vi "Fpga-Test-Harness.vi"() -> ()   [LabVIEW 2016]
uses:
  <vilib>/Platform/TimedLoop/XDataNode/timing_clust.ctl
  <vilib>/Platform/TimedLoop/XDataNode/nitl_modes.ctl
  <vilib>/Platform/TimedLoop/XDataNode/wakeup.ctl
  <vilib>/rvi/Emulation/niFpgaSctlEmulationGetInTimedLoop.vi
  <vilib>/rvi/Emulation/niFpgaEmulationReportErrorSimple.vi
  <vilib>/rvi/Emulation/niFpgaGetClockAttributes.vi
  <vilib>/rvi/Emulation/niFpgaCriticalErrorInLSC.vi
  <vilib>/rvi/interface/RandomDataEmulation/niFpgaRandomDataHandleErrors.vi
  <vilib>/rvi/Emulation/niFpgaEmulationIsFPGAContextNoSignature.vi
  <vilib>/rvi/errors/niFpgaSetErrorForExecOnDevCompSimple.vi
  <vilib>/rvi/eio/common/nirviEmuReportErrorAndStop.vi
  <vilib>/rvi/DataTransferAndStorage/Container/Common/niFpgaContainerGetUniqueNameForEmu.vi
  <vilib>/rvi/FIFO/Fifo_Resource/nirvififoEmulationSetSize.vi
  <vilib>/rvi/FIFO/Fifo_Resource/nirviFifoEmulationQueueMgr.vi
  <instcachedir>/0/nirviFifoEmulationQueueMgr_E5CAEC123FF24DC58D834DCA3CDAA9B5.lvgen/nirviFifoEmulationQueueMgr_E5CAEC123FF24DC58D834DCA3CDAA9B5_000.vi
  <vilib>/rvi/FIFO/Fifo_Resource/nirvififoEmulationDetermineInputValidOut.vi
  <vilib>/rvi/FIFO/Fifo_Resource/nirvififoEmulationCreateLock.vi
  <vilib>/rvi/Emulation/niFpgaProcessEmulError.vi
  <vilib>/rvi/FIFO/Fifo_Resource/nirvififoEmulationObtainLock.vi
  <vilib>/rvi/FIFO/Fifo_Resource/nirvififoEmulationReleaseLock.vi
  <vilib>/rvi/occurrence/nirviWaitOnOccurrenceBase.vi
  <vilib>/rvi/errors/nirviReportUnexpectedCaseInternalError.vi
  <vilib>/rvi/errors/nirviReportUnexpectedCaseInternalError (U32).vi
  <instcachedir>/0/nirviFifoEmulationQueueMgr_E5CAEC123FF24DC58D834DCA3CDAA9B5.lvgen/nirviFifoEmulationQueueMgr_E5CAEC123FF24DC58D834DCA3CDAA9B5_006.vi
  <vilib>/Utility/error.llb/Clear Errors.vi
  <vilib>/Platform/TimedLoop/XDataNode/XDataNode.xnode
  <vilib>/rvi/DataTransferAndStorage/Container/XNode/niFpgaContainer.xnode
  <vilib>/rvi/interface/RandomDataEmulation/nirviRandomDataFpgaReadWriteTemplate.vi
  <vilib>/rvi/FIFO/Fifo_Resource/nirvififoEmulationWrite.vi
  <vilib>/rvi/FIFO/Fifo_Resource/nirvififoEmulationRead.vi
  <vilib>/Platform/TimedLoop/XDataNode/XDNodeRunTimeDep.lvlib
panel:
  in  "Operating\nMode":enum16{"OrderBook"}(ring)
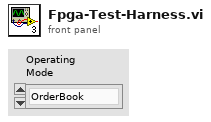
[diagram p1: front panel]
types:
  T1 = cluster{"Side":u16, "OrderRefNum":u64, "Price":u32, "Shares":u32}
  T2 = typedef "XDNodeRunTimeDep.lvlib/timing_clust.ctl" = cluster{"Expected End [f-1]":u64, "Actual End [f-1]":u64, "Finished Late? [f-1]":bool, "Expected End [i-1]":u64, "Actual End [i-1]":u64, "Finished Late? [i-1]":bool, "Expected Start [i]":u64, "Actual Start [i]":u64, "Expected Start [f]":u64, "Actual Start [f]":u64, "Source Name":string, "Structure Name":string, "Period":i64, "Deadline":i64, "Offset":i64, "Start":i64, "Priority":i32, "Timeout":i32, "Mode":T3, "Wakeup Reason":T4, "Error":errorcluster, "Source Type":string, "Secondary Source Type":string, "Global End Time":u64, "Global Start Time":u64, "Frame Duration":u64, "Iteration Duration":u64, "Assigned CPU":i32, "I/O Scan Engine Mode":u32}
  T3 = typedef "XDNodeRunTimeDep.lvlib/nitl_modes.ctl" = enum32{"No Change", "Process missed periods, maintain original phase", "Discard missed periods, maintain original phase", "Process missed periods, ignore original phase", "Discard missed periods, ignore original phase"}
  T4 = typedef "XDNodeRunTimeDep.lvlib/wakeup.ctl" = enum32{"Normal", "Aborted", "Asynchronous wakeup", "Timing source error", "Timed loop error", "Timeout"}
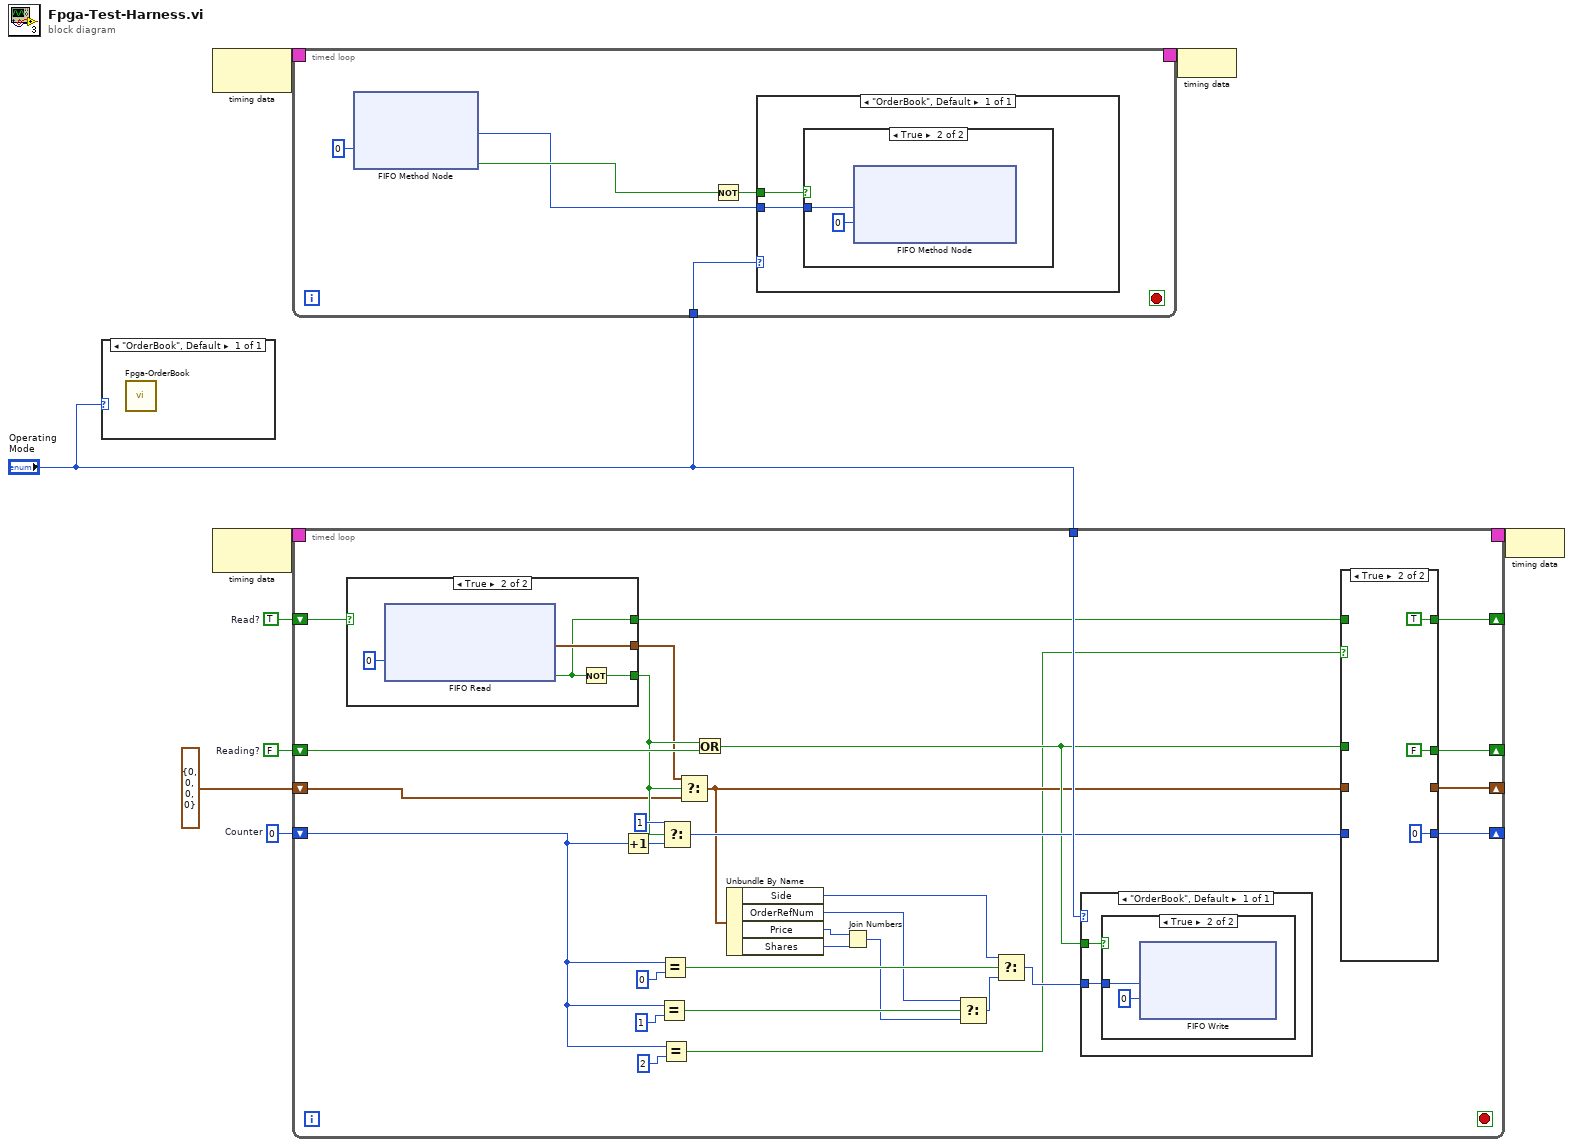
[diagram p0: block diagram]
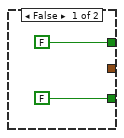
[diagram p3: hidden frame]
diagram:
  w3 = FALSE  # Reading?
  w4 = i16 0  # Counter
  w5 = TRUE  # Read?
  n1 = case shown="\"OrderBook\", Default" "Operating\nMode" {
    frame "OrderBook", Default {
      n2 = call "Fpga-OrderBook.vi"() -> ()  [unwired: 12 in]
    }
  }
  n3 = node-c288() -> (w9:T2)  [unwired: 1 in]
  n4 = node-c288() -> (w7:T2)  [unwired: 1 in]
  n5 = timed-loop {
    timing: w9 -> [_]
    timing-out: [_] -> w8
    tunnel: "Operating\nMode" -> [w10]
    stop <- _ stop-if-true
    n6 = xnode ("FIFO Method Node")("Timeout"=0) -> ("Element"=w11:u64, "Timed Out?"=w13:bool)  [unwired: 1 in, 1 out]
    n7 = Not(x=w13) -> (.not. x?=w12:bool)
    n8 = case shown="\"OrderBook\", Default" w10 {
      tunnel: w12 -> [w16]
      tunnel: w11 -> [w15]
      frame "OrderBook", Default {
        n9 = case shown="True" w16 {
          tunnel: w15 -> [_ w18]
          frame False {
          }
          frame True {
            n10 = xnode ("FIFO Method Node")("Element"=w18, "Timeout"=0) -> ()  [unwired: 1 in, 2 out]
          }
        }
      }
    }
  }
  n11 = timed-loop {
    timing: w7 -> [_]
    timing-out: [_] -> w6
    tunnel: "Operating\nMode" -> [w50]
    shift-right: [w47] -> _
    shift-left: w5 -> [w48]
    shift-right: [w45] -> _
    shift-left: w4 -> [w32]
    shift-right: [w43] -> _
    shift-left: w3 -> [w44]
    shift-right: [w37] -> _
    shift-left: T1 {"Side"=0, "OrderRefNum"=0, "Price"=0, "Shares"=0} ("Element") -> [w36]
    stop <- _ stop-if-true
    n12 = case shown="True" w48 {
      tunnel: [_ w62] -> w39
      tunnel: [FALSE ("Timed Out?") w61] -> w40
      tunnel: [FALSE w60] -> w46
      frame False {
      }
      frame True {
        n13 = xnode "FIFO Read"("Timeout"=0) -> ("Element"=w62:T1, "Timed Out?"=w60:bool)  [unwired: 1 in, 1 out]
        n14 = Not(x=w60) -> (.not. x?=w61:bool)
      }
    }
    n15 = Increment(x=w32) -> (x+1=w49:i16)
    n16 = Equal?(x=w32, y=i16 1) -> (x = y?=w27:bool)
    n17 = Equal?(x=w32, y=i16 0) -> (x = y?=w30:bool)
    n18 = Equal?(x=w32, y=i16 2) -> (x = y?=w21:bool)
    n19 = Select(t=i16 1, s=w40, f=w49) -> (s? t:f=w41:i16)
    n20 = Select(t=w39, s=w40, f=w36) -> (s? t:f=w31:T1)
    n21 = Or(x=w40, y=w44) -> (x .or. y?=w38:bool)
    n22 = Unbundle By Name(w31) -> ("Side"=w29:u16, "OrderRefNum"=w25:u64, "Price"=w24:u32, "Shares"=w23:u32)
    n23 = Join Numbers(hi=w24, lo=w23) -> ((hi.lo)=w22:u64)
    n24 = Select(t=w25, s=w27, f=w22) -> (s? t:f=w28:u64)
    n25 = Select(t=w29, s=w30, f=w28) -> (s? t:f=w26:u64)
    n26 = case shown="\"OrderBook\", Default" w50 {
      tunnel: w38 -> [w65]
      tunnel: w26 -> [w64]
      frame "OrderBook", Default {
        n27 = case shown="True" w65 {
          tunnel: w64 -> [_ w66]
          frame False {
          }
          frame True {
            n28 = xnode "FIFO Write"("Element"=w66, "Timeout"=0) -> ()  [unwired: 1 in, 2 out]
          }
        }
      }
    }
    n29 = case shown="True" w21 {
      tunnel: [w54 TRUE ("Timed Out?")] -> w47
      tunnel: w46 -> [w54 _]
      tunnel: w41 -> [w53 _]
      tunnel: [w53 i16 0 ("Counter")] -> w45
      tunnel: w38 -> [w52 _]
      tunnel: [w52 FALSE] -> w43
      tunnel: [w51 _] -> w37
      tunnel: w31 -> [w51 _]
      frame False {
      }
      frame True {
      }
    }
  }
  n30 = node-c288(w8) -> ()
  n31 = node-c288(w6) -> ()
